vi "Test Sequencing.vi"() -> ()   [LabVIEW 2013]
uses:
  Reusable/Sequence/SEQ/SEQ.lvclass
  State data/State Data.lvclass
  Data/cPAS Data.lvclass
  Data/cPAS Cell Data/cPAS Cell Data.lvclass
  CRDS/Data/cCRDS Data.lvclass
  State data/State Data.lvclass/State Data.ctl
  Builder/Cal Sequence Builder.lvclass
  Stability data/Stability Data.lvclass
  Reusable/Data/Array Data/Single 1-D/Single_Array.lvclass
  Reusable/Data/Double/Double.lvclass
  Data DVR/cPAS Data DVR.lvclass
  Reusable/Data/U16/U16.lvclass
  Associated data/Associated Data.lvclass
  Associated data/Associated Data.lvclass/Associated Data.ctl
  Builder/config data.ctl
  Data DVR/cPAS Data DVR.lvclass/cPAS Data DVR.ctl
  Reusable/Sequence/Sequence Factory/Sequence Builder.lvclass/Sequence Builder.ctl
  Builder/Cal Sequence Builder.lvclass/Cal Sequence Builder.ctl
  Reusable/Sequence/Sequence Factory/Accessors/Write Config Data.vi
  Builder/Write Stored State DVR.vi
  Reusable/Data/Write measTime.vi
  Reusable/PAS/Data/Cell/Write derived.vi
  Reusable/PAS/Data/Cell/Write houseKeeping.vi
  Reusable/PAS/Data/Main/Write CellData.vi
  Stability data/Set Data.vi
  <vilib>/Utility/file.llb/Write To Spreadsheet File (string).vi
  <vilib>/Utility/file.llb/Write To Spreadsheet File (DBL).vi
  <vilib>/Analysis/NI_AALBase.lvlib
panel:
  in  "O3 Stab Wait":dbl
  in  "Las Stab Wait":dbl=12.0
  out "RSE":dbl(graph)
  out "LRMS":T1(graph)
  in  "laserRMS":sgl=100.0
  in  "lRMS Noise":dbl=0.1
  out "IA 2":cluster{"Mean":dbl, "Error":dbl}[][](array[cluster])
  out "Extinction":cluster{"Mean":dbl, "Error":dbl}[][](array[cluster])
  in  "ext noise":dbl=0.1
  out "opt chart":T2(graph)={"[0]"=59.34970562369895, "[1]"=10.464575398396796, "[2]"=23.07416304904923, "[3]"=25.912577856467045, "[4]"=41.96548794471471, "[5]"=19.965941401620178, "[6]"=-0.44398511362477033, "[7]"=4.752794707465228, "[8]"=6.529862095577735, "[9]"=12.74107129055443}
  out "Qo2 Chart":dbl(graph)=62.38027713517588
  in  "O2 Step":i32=3
  in  "IA noise":dbl=0.1
  in  "Qo2 noise":dbl=0.01
  in  "scale":sgl[](array[numeric])=[3.0, 2.0, 1.0, 0.5]
  in  "b":dbl=11.0
  in  "m":dbl=2.3
  in  "IA":sgl[](array[numeric])=[115.0, 20.0, 45.0, 52.0, 83.0]
  in  "Set Qo2":dbl=250.0
  in  "Las Stab":cluster{"Error":sgl, "# of Obs":u16}={"Error"=0.05, "# of Obs"=15}
  in  "O3 Stab":cluster{"Error":sgl, "# of Obs":u16}={"Error"=0.05, "# of Obs"=10}
  in  "Qo2":sgl[](array[numeric])=[1.0, 0.75, 0.5, 0.25]
  in  "purge":dbl=10.0
  in  "zero":dbl=12.0
  in  "Autocal":bool=TRUE
  out "seqtime":dbl[][](array[numeric]) caption="Time"
  out "seqMsg":string[](array[string])=["1:09:27 PM\tValve to oxygen changed to TRUE.", "1:09:27 PM\tO2 flow set to 500.000000.", "1:09:32 PM\tMax orifice flow recorded.   Flow was 248.806366.", "1:09:42 PM\tStandard wait time elapsed.", "1:09:54 PM\tStandard wait time elapsed.", "1:09:55 PM\tLaser RMS stable in every cell. RSE Values: 0.000000\t0.000000\r\n", "1:09:55 PM\tSpeaker position changed to TRUE.", "1:09:55 PM\tO2 flow set to 248.806366.", "1:10:01 PM\tOzone stable in every cell.  Begin collecting data. RSE Values: 0.043430\t0.043108\t0.043108\t0.043537\t0.043537\t0.047428\t0.047428\t0.043882\t0.043882\t0.044978\t0.044978\t0.043616\t0.043616\t0.042956\r\n", "1:10:21 PM\tCollection step complete.", "1:10:21 PM\tO2 flow set to 186.604774.", "1:10:27 PM\tOzone stable in every cell.  Begin collecting data. RSE Values: 0.049616\t0.048562\t0.048562\t0.048143\t0.048143\t0.048496\t0.048678\t0.048678\t0.047656\t0.047656\t0.046716\t0.046716\t0.046716\r\n", "1:10:47 PM\tCollection step complete.", "1:10:47 PM\tO2 flow set to 124.403183.", "1:10:53 PM\tOzone stable in every cell.  Begin collecting data. RSE Values: 0.045074\t0.045269\t0.045269\t0.045371\t0.045371\t0.046657\t0.046657\t0.044803\t0.044803\t0.046626\t0.046626\t0.044248\t0.044248\t0.044248\r\n", "1:11:13 PM\tCollection step complete.", "1:11:13 PM\tO2 flow set to 62.201591.", "1:11:19 PM\tOzone stable in every cell.  Begin collecting data. RSE Values: 0.047075\t0.046939\t0.046939\t0.049594\t0.049594\t0.046739\t0.046655\t0.046655\t0.046655\t0.048990\t0.048989\t0.048989\t0.048989\r\n", "1:11:39 PM\tCollection step complete.", "1:11:39 PM\tData displayed!", "1:11:39 PM\tSpeaker position changed to FALSE.", "1:11:39 PM\tValve to oxygen changed to FALSE.", "1:11:39 PM\tO2 flow set to 0.000000.", "1:11:49 PM\tStandard wait time elapsed.", "1:12:02 PM\tStandard wait time elapsed."] caption="Messages"
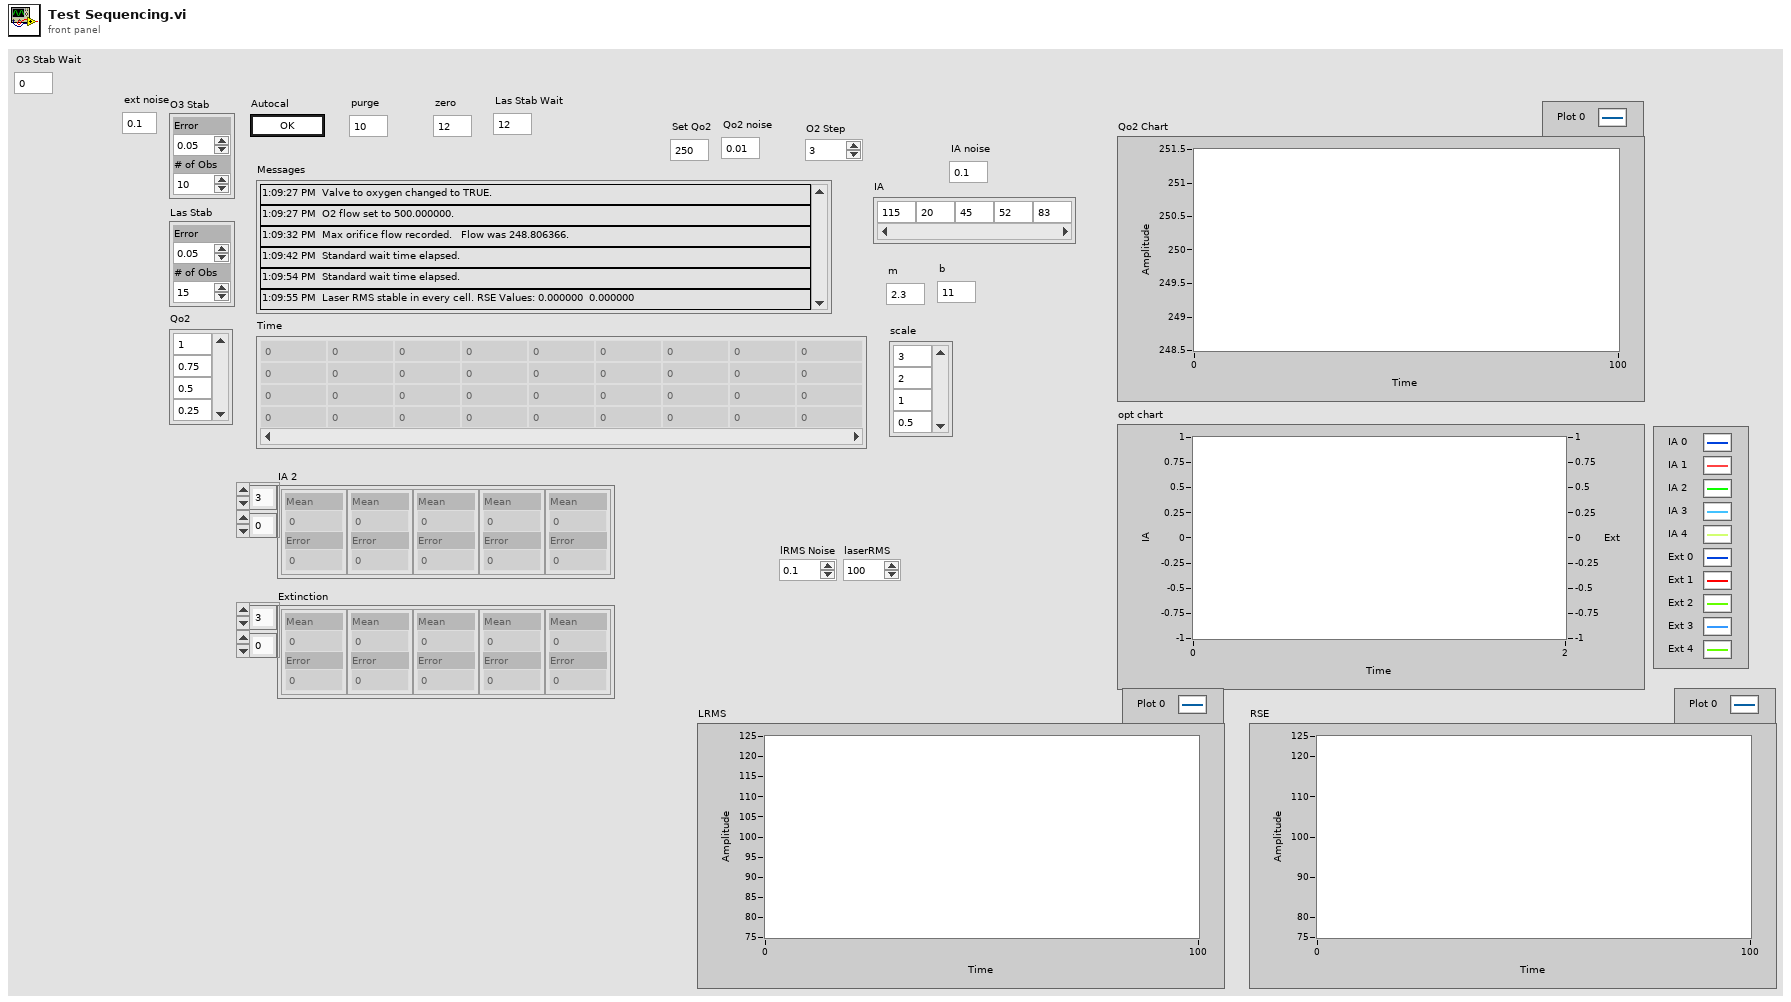
[diagram p1: front panel]
types:
  T1 = cluster{"[0]":dbl, "[1]":dbl, "[2]":dbl, "[3]":dbl, "[4]":dbl}
  T2 = cluster{"[0]":dbl, "[1]":dbl, "[2]":dbl, "[3]":dbl, "[4]":dbl, "[5]":dbl, "[6]":dbl, "[7]":dbl, "[8]":dbl, "[9]":dbl}
  T3 = cluster{"Stored State":refnum<class "State Data.lvclass">[], "pointer to data":i32}
  T4 = typedef "Cal Sequence Builder.lvclass/config data.ctl" = enum16{"purge time", "zero time", "qo2", "o3 stability", "laser stability", "pas state dvr", "collection observations", "associated cells", "crds state dvr", "Init Filter State"}
  T5 = cluster{"f0":sgl, "IA":sgl, "Q":sgl, "max":dbl[], "deltaPhi":dbl, "tau":dbl, "noiseLim":dbl, "ext":dbl}
  T6 = cluster{"T":sgl, "TRH":sgl, "RH":sgl, "laserRMS":sgl}
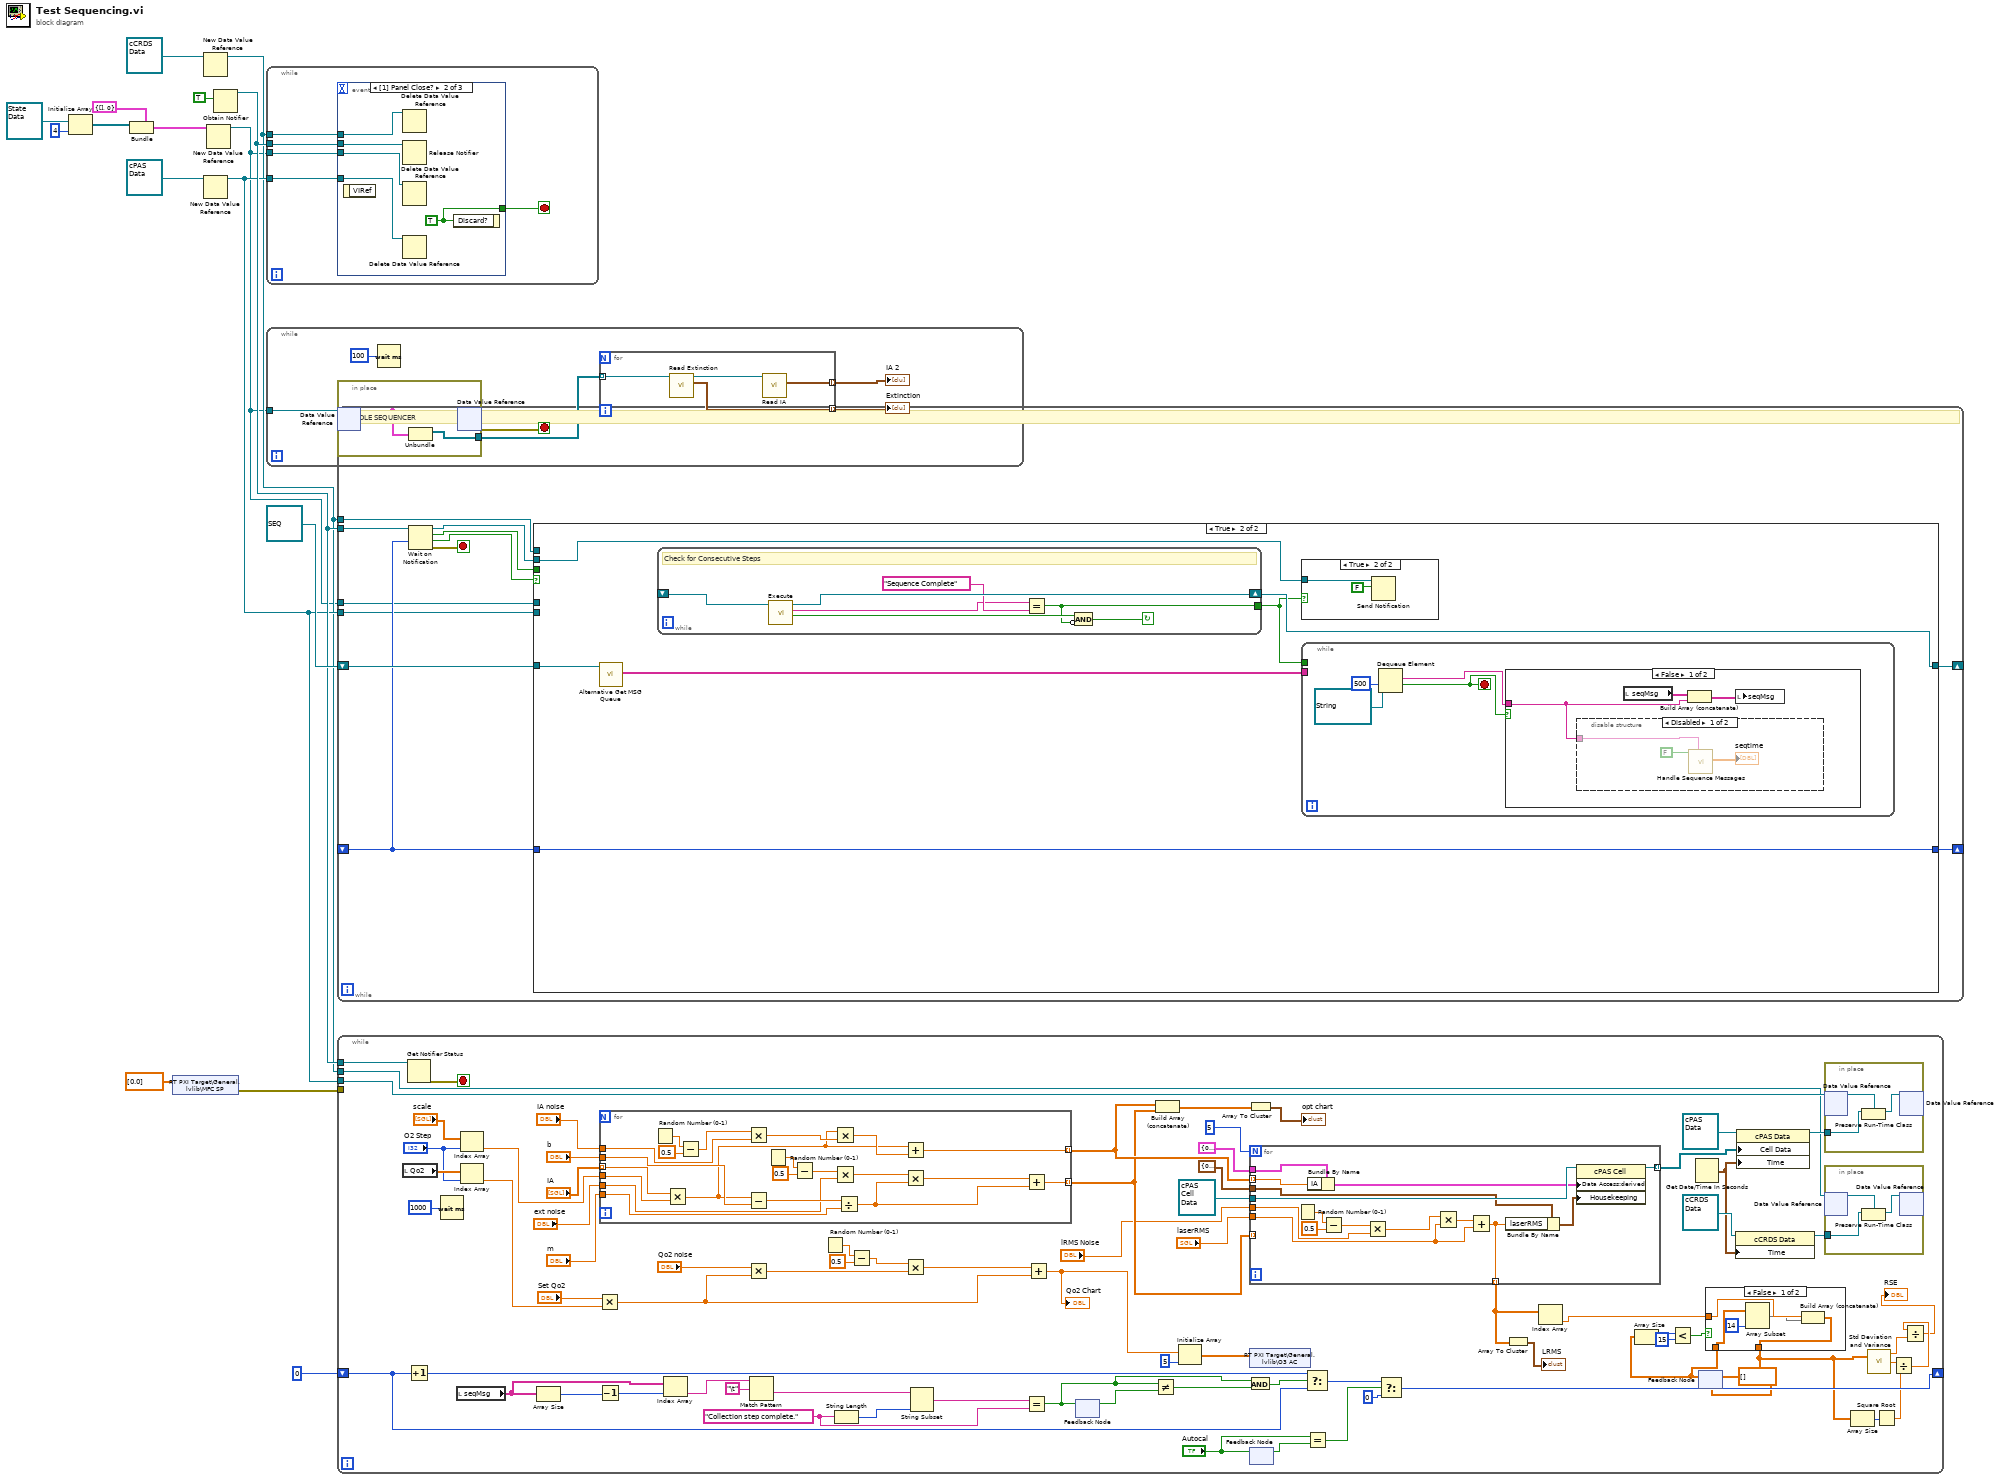
[diagram p0: block diagram]
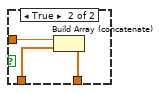
[diagram p2: hidden frame]
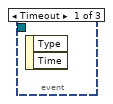
[diagram p3: hidden frame]
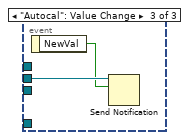
[diagram p4: hidden frame]
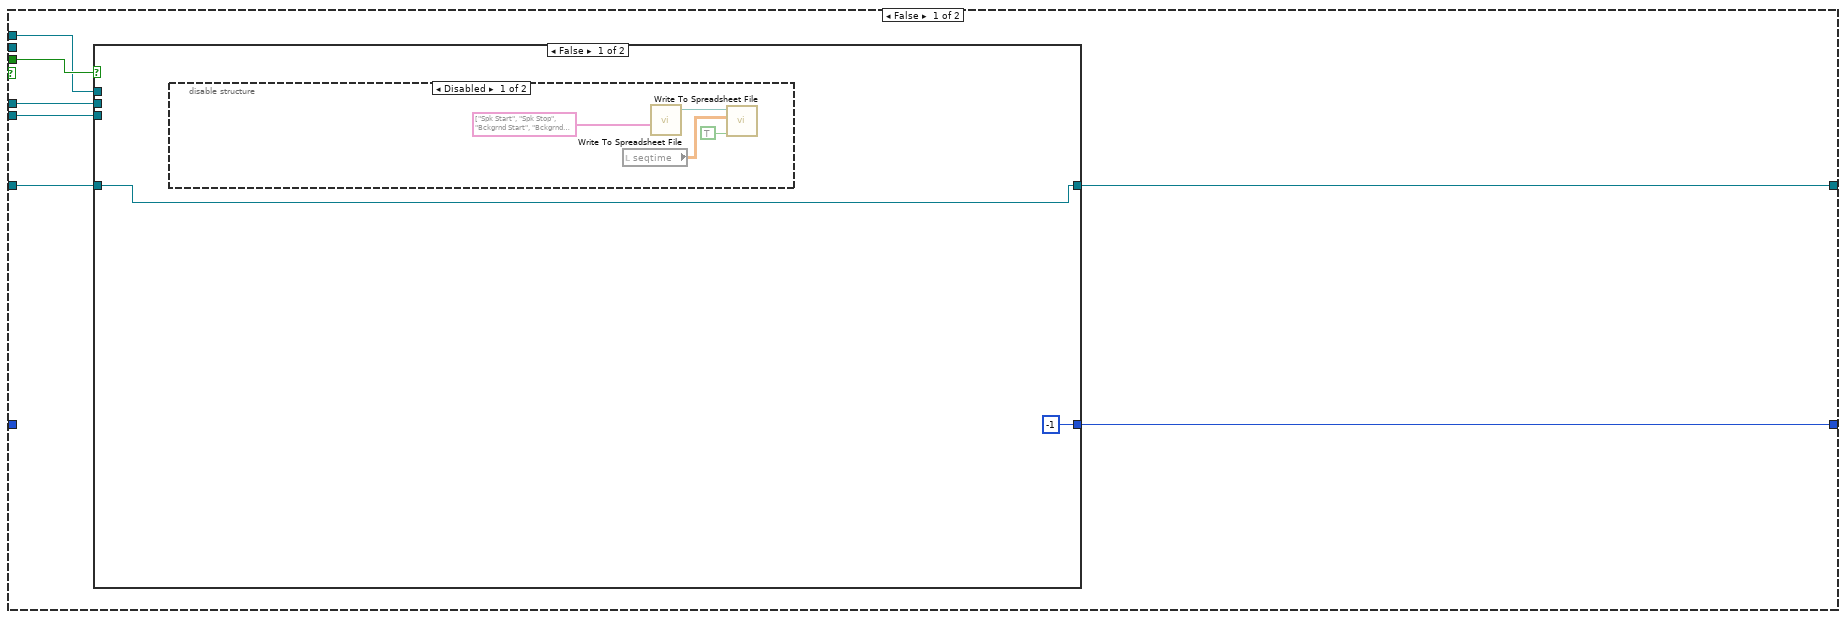
[diagram p5: hidden frame]
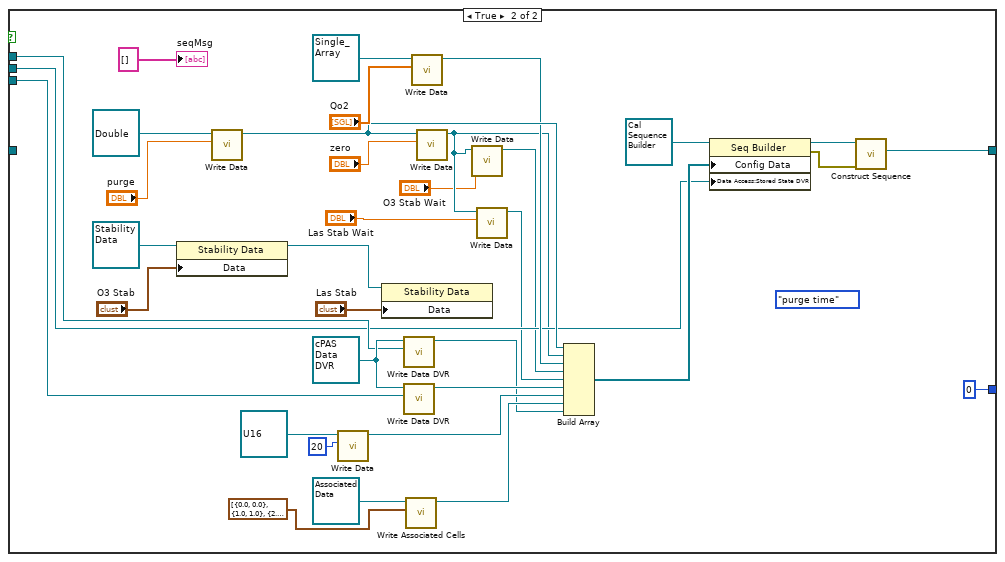
[diagram p7: hidden frame]
diagram:
  n1 = Initialize Array(refnum<class "State Data.lvclass"> refnum ("State Data"), 4 ("dimension size")) -> (w3:refnum<class "State Data.lvclass">[])
  n2 = Bundle(cluster=T3 {"Stored State"=[], "pointer to data"=0} ("Data and Pointer"), "Stored State"=w3) -> (w2:T3)  [unwired: 1 in]
  n3 = shared-variable "RT PXI Target\\General.lvlib\\MFC SP"(sgl[] [0.0] ("MFC SP")) -> (error out=w10:errorcluster)  [unwired: 1 in]
  n4 = New Data Value Reference(data value=refnum<class "cCRDS Data.lvclass"> refnum ("cCRDS Data")) -> (data value reference=w8:refnum<data-value>)  [unwired: 1 in, 1 out]
  n5 = New Data Value Reference(data value=refnum<class "cPAS Data.lvclass"> refnum ("cPAS Data")) -> (data value reference=w9:refnum<data-value>)  [unwired: 1 in, 1 out]
  n6 = New Data Value Reference(data value=w2) -> (data value reference=w7:refnum<data-value>)  [unwired: 1 in, 1 out]
  n7 = Obtain Notifier(notification data type=TRUE) -> (notifier out=w14:refnum<notifier>)  [unwired: 3 in, 2 out]
  n8 = while {
    tunnel: w14 -> [w20]
    tunnel: w9 -> [w19]
    tunnel: w8 -> [w18]
    tunnel: w7 -> [w17]
    stop <- w21 stop-if-true
    n9 = event shown="[1] Panel Close?" {
      selector: _ -> [_ _ _]
      dyn-events: _ -> [_ _ _]
      timeout: _ -> [_ _ _]
      tunnel: [_ w26 _] -> w21
      tunnel: w20 -> [_ w25 w28]
      tunnel: w19 -> [_ w24 _]
      tunnel: w18 -> [_ w23 _]
      tunnel: w17 -> [_ w22 _]
      event Timeout {
        n10 = event-data() -> ()  [unwired: 1 in, 2 out]
      }
      event Panel Close? {
        w26 = TRUE ("Discard?")
        n11 = event-data() -> ()  [unwired: 1 in, 1 out]
        n12 = Delete Data Value Reference(data value reference=w23) -> ()  [unwired: 1 in, 2 out]
        n13 = Release Notifier(notifier=w25) -> ()  [unwired: 2 in, 3 out]
        n14 = Delete Data Value Reference(data value reference=w22) -> ()  [unwired: 1 in, 2 out]
        n15 = Delete Data Value Reference(data value reference=w24) -> ()  [unwired: 1 in, 2 out]
        n16 = event-data("Discard?"=w26) -> ()  [unwired: 1 in, 1 out]
      }
      event "Autocal": Value Change {
        n17 = event-data() -> ("NewVal"=w27:bool)  [unwired: 1 in]
        n18 = Send Notification(notification=w27, notifier=w28) -> ()  [unwired: 1 in, 2 out]
      }
    }
  }
  n19 = while {
    tunnel: w7 -> [w34]
    stop <- w33 stop-if-true
    n20 = in-place {
      in-place-border: [w40] -> w32
      n21 = in-place-dvr #1(w34) -> (w39:T3)  [unwired: 1 out]
      n22 = Unbundle(w39) -> ("Stored State"=w40:refnum<class "State Data.lvclass">[])  [unwired: 1 out]
      n23 = in-place-dvr #1(w39) -> (w33:errorcluster)  [unwired: 1 out]
    }
    n24 = Wait (ms)(milliseconds to wait=u32 100) -> ()  [unwired: 1 out]
    n25 = for {
      tunnel: w32 -> [w38] mode=indexing
      tunnel: [w36] -> w31 mode=indexing
      tunnel: [w35] -> w30 mode=indexing
      n26 = call "Read Extinction.vi"("State Data in"=w38) -> ("Extinction"=w36:cluster{"Mean":dbl, "Error":dbl}[], "State Data out"=w37:refnum<class "State Data.lvclass">)  [unwired: 8 in, 1 out]
      n27 = call "Read IA.vi"("State Data in"=w37) -> ("IA"=w35:cluster{"Mean":dbl, "Error":dbl}[])  [unwired: 8 in, 2 out]
    }
    "Extinction" <- w31
    "IA 2" <- w30
  }
  n28 = while {
    shift-right: [w52] -> _
    shift-left: _ -> [w48]
    shift-right: [w50] -> _
    shift-left: refnum<class "SEQ.lvclass"> refnum ("Sequence Composition:SEQ") -> [w51]
    tunnel: w14 -> [w44]
    tunnel: w9 -> [w43]
    tunnel: w8 -> [w42]
    tunnel: w7 -> [w41]
    stop <- w49 stop-if-true
    # "HANDLE SEQUENCER"
    n29 = Wait on Notification(notifier=w44, timeout in ms (-1)=w48) -> (notifier out=w45:refnum<notifier>, notification=w46:bool, timed out?=w47:bool, error out=w49:errorcluster)  [unwired: 2 in]
    n30 = case shown="True" w47 {
      tunnel: w46 -> [w57 _]
      tunnel: [w59 w105] -> w52
      tunnel: w51 -> [w56 w102]
      tunnel: [w58 w106] -> w50
      tunnel: w48 -> [_ w105]
      tunnel: w45 -> [_ w104]
      tunnel: w43 -> [w55 _]
      tunnel: w42 -> [w54 _]
      tunnel: w41 -> [w53 _]
      frame False {
        n31 = case shown="False" w57 {
          tunnel: [w60 w98] -> w58
          tunnel: [-1 0 ("t")] -> w59
          tunnel: w56 -> [w60 _]
          tunnel: w55 -> [_ w81]
          tunnel: w54 -> [_ w80]
          tunnel: w53 -> [_ w71]
          frame False {
            n32 = disable-structure shown="Disabled" {
              frame Disabled {
                n33 = local read "seqtime"() -> (w63:dbl[][])
                n34 = call-poly <vilib>:"Write To Spreadsheet File.vi"("1D data"=string[] ["Spk Start", "Spk Stop", "Bckgrnd Start", "Bckgrnd Stop", "Sample Start", "Sample Stop", "Cal Start", "Cal Stop", "Cal #"]) -> ("new file path (Not A Path if cancelled)"=w64:path)  [unwired: 7 in]
                n35 = call-poly <vilib>:"Write To Spreadsheet File.vi"("append to file? (new file:F)"=TRUE, "2D data"=w63, "file path (dialog if empty)"=w64) -> ()  [unwired: 5 in, 1 out]
              }
              frame Enabled {
              }
            }
          }
          frame True {
            (unwired) config_data."purge time" ("config data")
            w82 = refnum<class "cPAS Data DVR.lvclass"> refnum ("cPAS Data DVR.lvclass")
            n36 = property class="Stability Data"(reference=refnum<class "Stability Data.lvclass"> refnum ("Stability Data"), "Data"="O3 Stab") -> (reference out=w83:refnum<class "Stability Data.lvclass">)  [unwired: 1 in, 1 out]
            n37 = call "Write Data.vi"("Data"="purge", "Double in"=refnum<class "Double.lvclass"> refnum ("Base Data Class.lvlib:Double.lvclass")) -> ("Double out"=w87:refnum<class "Double.lvclass">)  [unwired: 8 in, 1 out]
            n38 = call "Write Data.vi"("Data"=u16 20, "U16 in"=refnum<class "U16.lvclass"> refnum ("Base Data Class.lvlib:U16")) -> ("U16 out"=w74:refnum<class "U16.lvclass">)  [unwired: 8 in, 1 out]
            n39 = property class="Stability Data"(reference=w83, "Data"="Las Stab") -> ()  [unwired: 1 in, 2 out]
            n40 = call "Write Data DVR.vi"("Data DVR"=w80, "cPAS Data DVR in"=w82) -> ("cPAS Data DVR out"=w72:refnum<class "cPAS Data DVR.lvclass">)  [unwired: 8 in, 1 out]
            n41 = call "Write Data DVR.vi"("Data DVR"=w81, "cPAS Data DVR in"=w82) -> ("cPAS Data DVR out"=w79:refnum<class "cPAS Data DVR.lvclass">)  [unwired: 8 in, 1 out]
            n42 = call "Write Associated Cells.vi"("Associated Cells"=cluster{"PAS":dbl, "CRD":dbl}[] [{"PAS"=0.0, "CRD"=0.0}, {"PAS"=1.0, "CRD"=1.0}, {"PAS"=2.0, "CRD"=2.0}, {"PAS"=3.0, "CRD"=3.0}, {"PAS"=4.0, "CRD"=4.0}], "Associated Data in"=refnum<class "Associated Data.lvclass"> refnum ("Associated Data.lvclass")) -> ("Associated Data out"=w73:refnum<class "Associated Data.lvclass">)  [unwired: 8 in, 1 out]
            n43 = call "Write Data.vi"("Data"="Qo2", "Single_Array in"=refnum<class "Single_Array.lvclass"> refnum ("Base Data Class.lvlib:Single_Array.lvclass")) -> ("Single_Array out"=w86:refnum<class "Single_Array.lvclass">)  [unwired: 8 in, 1 out]
            n44 = call "Write Data.vi"("Data"="zero", "Double in"=w87) -> ("Double out"=w69:refnum<class "Double.lvclass">)  [unwired: 8 in, 1 out]
            n45 = call "Write Data.vi"("Data"="O3 Stab Wait", "Double in"=w69) -> ("Double out"=w67:refnum<class "Double.lvclass">)  [unwired: 8 in, 1 out]
            n46 = call "Write Data.vi"("Data"="Las Stab Wait", "Double in"=w69) -> ("Double out"=w66:refnum<class "Double.lvclass">)  [unwired: 8 in, 1 out]
            n47 = Build Array(w87, w69, w86, w67, w66, w79, w74, w73, w72) -> (w85:refnum<class "Data.lvclass">[])
            n48 = property class="Seq Builder"(reference=refnum<class "Cal Sequence Builder.lvclass"> refnum ("Cal Sequence Builder in"), "Config Data"=w85, "Data Access:Stored State DVR"=w71) -> (reference out=w96:refnum<class "Cal Sequence Builder.lvclass">, error out=w95:errorcluster)  [unwired: 1 in]
            n49 = call-dynamic "Construct Sequence.vi"("error in"=w95, "Cal Sequence Builder in"=w96) -> ("New Sequence"=w98:refnum<class "SEQ.lvclass">)  [unwired: 7 in, 2 out]
            "seqMsg" <- string[] [] ("Messages")
          }
        }
      }
      frame True {
        n50 = call "Alternative Get MSG Queue.vi"("SEQ in"=w102) -> ("seqMsg"=w101:string[])  [unwired: 9 in, 1 out]
        n51 = while {
          shift-right: [w112] -> w106
          shift-left: _ -> [w113]
          tunnel: [w107] -> w103
          stop <- w108 continue-if-true
          # "Check for Consecutive Steps"
          n52 = call-dynamic "Execute.vi"("SEQ in"=w113) -> ("Next Step?"=w109:bool, "MSG"=w110:string, "SEQ out"=w112:refnum<class "SEQ.lvclass">)  [unwired: 7 in, 1 out]
          n53 = Equal?(x=w110, y="Sequence Complete" ("t")) -> (x = y?=w107:bool)
          n54 = Compound Arithmetic op=AND(w109, invert w107) -> (w108:bool)
        }
        n55 = case shown="True" w103 {
          tunnel: w104 -> [_ w115]
          frame False {
          }
          frame True {
            n56 = Send Notification(notification=FALSE, notifier=w115) -> ()  [unwired: 1 in, 2 out]
          }
        }
        n57 = while {
          tunnel: w101 -> [_]
          tunnel: w103 -> [_]
          stop <- w117 stop-if-true
          n58 = Dequeue Element(queue=refnum<queue> refnum, timeout in ms (-1)=500) -> (element=w118:string, timed out?=w117:bool)  [unwired: 1 in, 2 out]
          n59 = case shown="False" w117 {
            tunnel: w118 -> [w120 _]
            frame False {
              n60 = disable-structure shown="Disabled" {
                disable-tunnel: w120 -> [w125 _]
                frame Disabled {
                  n61 = call "Handle Sequence Messages.vi"("MSG"=w125, "Init?"=FALSE) -> ("Array out"=→"seqtime":dbl[][])  [unwired: 7 in, 2 out]
                }
                frame Enabled {
                }
              }
              n62 = local read "seqMsg"() -> (w121:string[])
              n63 = Build Array (concatenate)(w121, w120) -> (w122:string[])
              n64 = local write "seqMsg"(w122) -> ()
            }
            frame True {
            }
          }
        }
      }
    }
  }
  n65 = while {
    tunnel: w14 -> [w203]
    tunnel: w9 -> [w175]
    tunnel: w8 -> [w173]
    tunnel: w10 -> [_]
    shift-right: [w146] -> _
    shift-left: 0 -> [w150]
    stop <- w202 stop-if-true
    w156 = "Collection step complete."
    n66 = local read "Qo2"() -> (w165:sgl[])
    n67 = Get Notifier Status(notifier=w203) -> (error out=w202:errorcluster)  [unwired: 1 in, 4 out]
    n68 = Increment(x=w150) -> (x+1=w151:i32)
    n69 = Wait (ms)(milliseconds to wait=u32 1000) -> ()  [unwired: 1 out]
    n70 = local read "seqMsg"() -> (w164:string[])
    n71 = Index Array(array="scale", index="O2 Step") -> (element=w190:sgl)
    n72 = Index Array(array=w165, index="O2 Step") -> (element=w180:sgl)
    n73 = Array Size(array=w164) -> (size(s)=w163:i32)
    n74 = Multiply(x="Set Qo2", y=w180) -> (x*y=w179:dbl)
    n75 = Decrement(x=w163) -> (x-1=w162:i32)
    n76 = for {
      tunnel: w190 -> [w238]
      tunnel: "IA" -> [w228] mode=indexing
      tunnel: "IA noise" -> [w234]
      tunnel: [w231] -> w177 mode=indexing
      tunnel: "b" -> [w227]
      tunnel: "m" -> [w225]
      tunnel: "ext noise" -> [w223]
      tunnel: [w219] -> w171 mode=indexing
      n77 = Random Number (0-1)() -> (number: 0 to 1=w236:dbl)
      n78 = Multiply(x=w228, y=w238) -> (x*y=w218:sgl)
      n79 = Subtract(x=w236, y=0.5) -> (x-y=w237:dbl)
      n80 = Multiply(x=w237, y=w234) -> (x*y=w233:dbl)
      n81 = Subtract(x=w218, y=w227) -> (x-y=w226:dbl)
      n82 = Random Number (0-1)() -> (number: 0 to 1=w229:dbl)
      n83 = Subtract(x=w229, y=0.5) -> (x-y=w224:dbl)
      n84 = Multiply(x=w218, y=w233) -> (x*y=w232:dbl)
      n85 = Multiply(x=w224, y=w223) -> (x*y=w222:dbl)
      n86 = Divide(x=w226, y=w225) -> (x/y=w220:dbl)
      n87 = Add(x=w218, y=w232) -> (x+y=w231:dbl)
      n88 = Multiply(x=w222, y=w220) -> (x*y=w221:dbl)
      n89 = Add(x=w221, y=w220) -> (x+y=w219:dbl)
    }
    n90 = Index Array(array=w164, index=w162) -> (element=w161:string)
    n91 = Multiply(x="Qo2 noise", y=w179) -> (x*y=w193:dbl)
    n92 = Match Pattern(string=w161, regular expression="\t") -> (after substring=w159:string)  [unwired: 1 in, 3 out]
    n93 = Random Number (0-1)() -> (number: 0 to 1=w196:dbl)
    n94 = String Length(string=w156) -> (length=w158:i32)
    n95 = Subtract(x=w196, y=0.5) -> (x-y=w192:dbl)
    n96 = Multiply(x=w192, y=w193) -> (x*y=w191:dbl)
    n97 = String Subset(string=w159, length (rest)=w158) -> (substring=w157:string)  [unwired: 1 in]
    n98 = Equal?(x=w157, y=w156) -> (x = y?=w153:bool)
    n99 = Add(x=w191, y=w179) -> (x+y=w169:dbl)
    "Qo2 Chart" <- w169
    n100 = feedback-in #2(w153) -> ()
    n101 = feedback #2() -> (w155:bool)  [unwired: 1 in]
    n102 = Not Equal?(x=w153, y=w155) -> (x != y?=w154:bool)
    n103 = Build Array (concatenate)(w177, w171) -> (w184:dbl[])
    n104 = Initialize Array(w169, 5 ("dimension size")) -> (w167:dbl[])
    n105 = Array To Cluster(array=w184) -> (cluster=→"opt chart":T2)
    n106 = And(x=w153, y=w154) -> (x .and. y?=w152:bool)
    n107 = for {
      N: 5 -> [_]
      tunnel: refnum<class "cPAS Cell Data.lvclass"> refnum ("cPAS Cell") -> [w253]
      tunnel: [w252] -> w182 mode=indexing
      tunnel: T6 {"T"=0.0, "TRH"=0.0, "RH"=0.0, "laserRMS"=100.0} ("Housekeeping") -> [w241]
      tunnel: w177 -> [w250] mode=indexing
      tunnel: T5 {"f0"=0.0, "IA"=0.0, "Q"=0.0, "max"=[], "deltaPhi"=0.0, "tau"=0.0, "noiseLim"=0.0, "ext"=0.0} ("derived") -> [w251]
      tunnel: w171 -> [_] mode=indexing
      tunnel: "lRMS Noise" -> [w245]
      tunnel: "laserRMS" -> [w242]
      tunnel: [w239] -> w139 mode=indexing
      n108 = Random Number (0-1)() -> (number: 0 to 1=w248:dbl)
      n109 = Bundle By Name(cluster=w251, "IA"=w250) -> (w249:T5)
      n110 = Subtract(x=w248, y=0.5) -> (x-y=w246:dbl)
      n111 = Multiply(x=w246, y=w245) -> (x*y=w244:dbl)
      n112 = Multiply(x=w244, y=w242) -> (x*y=w243:dbl)
      n113 = Add(x=w243, y=w242) -> (x+y=w239:dbl)
      n114 = Bundle By Name(cluster=w241, "laserRMS"=w239) -> (w240:T6)
      n115 = property class="cPAS Cell"(reference=w253, "Data Access:derived"=w249, "Housekeeping"=w240) -> (reference out=w252:refnum<class "cPAS Cell Data.lvclass">)  [unwired: 1 in, 1 out]
    }
    n116 = shared-variable "RT PXI Target\\General.lvlib\\O3 AC"(w167) -> ()  [unwired: 1 in, 1 out]
    n117 = feedback-in #3("Autocal") -> ()
    n118 = feedback #3() -> (w149:bool)  [unwired: 1 in]
    n119 = Select(t=w151, s=w152, f=w150) -> (s? t:f=w143:i32)
    n120 = Equal?(x="Autocal", y=w149) -> (x = y?=w148:bool)
    n121 = Select(t=w143, s=w148, f=0) -> (s? t:f=w146:i32)
    n122 = Array To Cluster(array=w139) -> (cluster=→"LRMS":T1)
    n123 = Index Array(array=w139) -> (element=w134:dbl)  [unwired: 1 in]
    n124 = Get Date/Time In Seconds() -> (seconds since 1Jan1904=w166:timestamp)
    n125 = feedback #4(dbl[] []) -> (w133:dbl[])
    n126 = Array Size(array=w133) -> (size(s)=w137:i32)
    n127 = Less?(x=w137, y=15) -> (x < y?=w135:bool)
    n128 = case shown="False" w135 {
      tunnel: w134 -> [w207 w211]
      tunnel: w133 -> [w208 w210]
      tunnel: [w205 w209] -> w132
      frame False {
        n129 = Array Subset(array=w208, length=14) -> (w206:dbl[])  [unwired: 1 in]
        n130 = Build Array (concatenate)(w207, w206) -> (w205:dbl[])
      }
      frame True {
        n131 = Build Array (concatenate)(w211, w210) -> (w209:dbl[])
      }
    }
    n132 = feedback-in #4(w132) -> ()
    n133 = property class="cCRDS Data"(reference=refnum<class "cCRDS Data.lvclass"> refnum ("cCRDS Data"), "Time"=w166) -> (reference out=w170:refnum<class "cCRDS Data.lvclass">)  [unwired: 1 in, 1 out]
    n134 = property class="cPAS Data"(reference=refnum<class "cPAS Data.lvclass"> refnum ("cPAS Data"), "Cell Data"=w182, "Time"=w166) -> (reference out=w174:refnum<class "cPAS Data.lvclass">)  [unwired: 1 in, 1 out]
    n135 = in-place {
      in-place-border: w174 -> [w215]
      n136 = in-place-dvr #5(w175) -> (w217:refnum<class "cPAS Data.lvclass">)  [unwired: 1 out]
      n137 = Preserve Run-Time Class(object in=w215, 2:w217) -> (object out=w216:refnum<class "cPAS Data.lvclass">)  [unwired: 1 in, 1 out]
      n138 = in-place-dvr #5(w216) -> ()  [unwired: 2 out]
    }
    n139 = in-place {
      in-place-border: w170 -> [w212]
      n140 = in-place-dvr #6(w173) -> (w214:refnum<class "cCRDS Data.lvclass">)  [unwired: 1 out]
      n141 = Preserve Run-Time Class(object in=w212, 2:w214) -> (object out=w213:refnum<class "cCRDS Data.lvclass">)  [unwired: 1 in, 1 out]
      n142 = in-place-dvr #6(w213) -> ()  [unwired: 2 out]
    }
    n143 = Array Size(array=w132) -> (size(s)=w131:i32)
    n144 = call <vilib>:"Std Deviation and Variance.vi"("X"=w132) -> ("mean"=w128:dbl, "standard deviation"=w130:dbl)  [unwired: 1 in, 1 out]
    n145 = Square Root(x=w131) -> (sqrt(x)=w129:dbl)
    n146 = Divide(x=w130, y=w129) -> (x/y=w127:dbl)
    n147 = Divide(x=w127, y=w128) -> (x/y=→"RSE":dbl)
  }
